vi "Start Needed uServices.vi"(8 "error in (no error)":errorcluster, 11 "Tamer in":refnum<class "Tamer.lvclass">) -> (0 "error out":errorcluster, 2 "All online?":bool, 3 "Tamer out":refnum<class "Tamer.lvclass">)   [LabVIEW 2020, in "TALOS.lvlib" / "Tamer.lvlib" / "Tamer.lvclass"]
uses:
  Tamer.lvclass
  Tamer.lvclass/Tamer.ctl
  Support VIs/Global Memory.vi
  Interfaces/FPGA Interface/FPGA Interface.lvclass
  TALOS.lvlib
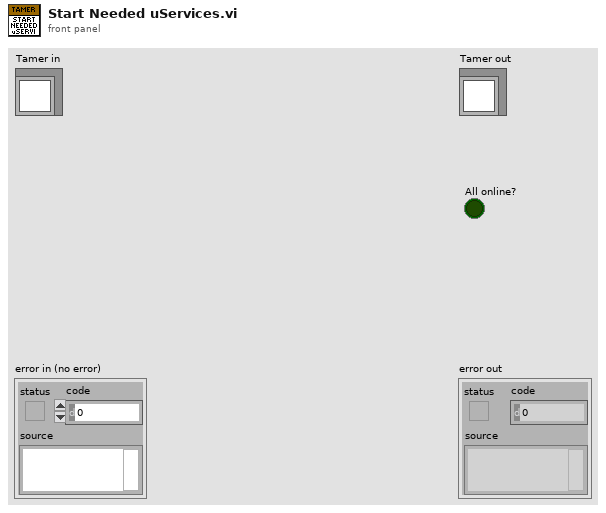
[diagram p1: front panel]
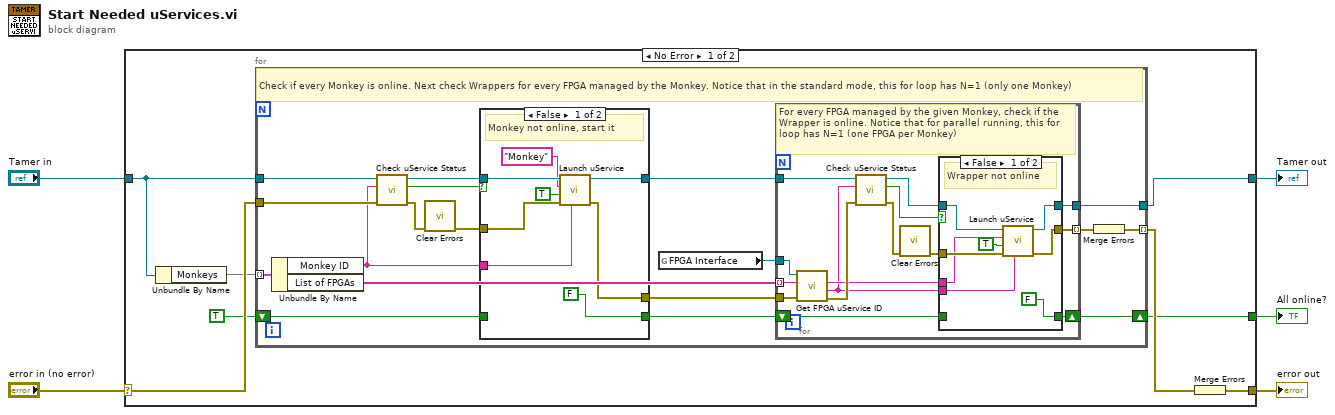
[diagram p0: block diagram]
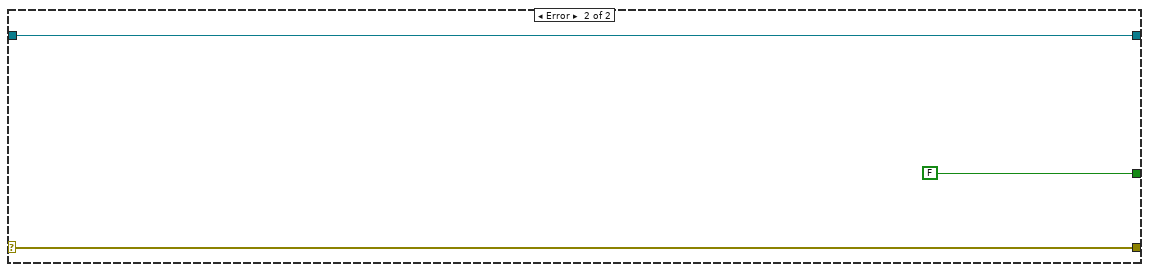
[diagram p4: hidden frame]
diagram:
  n1 = case shown="No Error" "error in (no error)" {
    selector: "error in (no error)" -> [w12 w71]
    tunnel: [w6 w71] -> w4
    tunnel: [w9 w70] -> w2
    tunnel: "Tamer in" -> [w10 w70]
    tunnel: [w7 FALSE] -> w1
    frame No Error {
      n2 = Unbundle By Name(w10) -> ("Monkeys"=w11:map{string, string[]})
      n3 = for {
        tunnel: w11 -> [w30] mode=indexing
        tunnel: w12 -> [w28]
        tunnel: w10 -> [w24]
        tunnel: [w21] -> w9
        tunnel: [w14] -> w13 mode=indexing
        shift-right: [w18] -> w7
        shift-left: TRUE -> [w20]
        # "Check if every Monkey is online. Next check Wrappers for every FPGA managed by the Monkey. Notice that in the standard mode, this for loop has N=1 (only one Monkey)"
        n4 = Unbundle By Name(w30) -> ("Monkey ID"=w25:string, "List of FPGAs"=w31:string[])
        n5 = call-dynamic "Check uService Status.vi"("error in (no error)"=w28, "uService ID"=w25, "Father of all uServices in"=w24) -> ("error out"=w29:errorcluster, "Online?"=w27:bool, "Father of all uServices out"=w26:refnum<class "Tamer.lvclass">)  [unwired: 5 in, 1 out]
        n6 = call <vilib>:"Clear Errors.vi"("error in (no error)"=w29) -> ("error out"=w23:errorcluster)  [unwired: 5 in, 1 out]
        n7 = case shown="False" w27 {
          tunnel: w26 -> [w38 w42]
          tunnel: w25 -> [w33 _]
          tunnel: [w37 w42] -> w22
          tunnel: w23 -> [w36 w41]
          tunnel: [w35 w41] -> w16
          tunnel: w20 -> [_ w40]
          tunnel: [FALSE w40] -> w19
          frame False {
            # "Monkey not online, start it"
            n8 = call-dynamic "Launch uService.vi"("uService ID (optional)"=w33, "error in (no error)"=w36, "GUI?"=TRUE, "Class Name"="Monkey", "Father of all uServices in"=w38) -> ("error out"=w35:errorcluster, "Father of all uServices out"=w37:refnum<class "Tamer.lvclass">)  [unwired: 5 in]
          }
          frame True {
            # "Monkey already online"
          }
        }
        n9 = global read "Global Memory.vi" "FPGA Interface"() -> (w17:refnum<class "FPGA Interface.lvclass">)
        n10 = for {
          tunnel: w31 -> [w47] mode=indexing
          tunnel: w22 -> [w57]
          tunnel: [w52] -> w21
          tunnel: [w51] -> w15 mode=indexing
          shift-right: [w49] -> w18
          shift-left: w19 -> [w50]
          tunnel: w17 -> [w48]
          tunnel: w16 -> [w46]
          # "For every FPGA managed by the given Monkey, check if the Wrapper is online. Notice that for parallel running, this for loop has N=1 (one FPGA per Monkey)"
          n11 = call-dynamic "Get FPGA uService ID.vi"("error in"=w46, "FPGA Name"=w47, "FPGA Interface"=w48) -> ("error out"=w45:errorcluster, "uService ID"=w43:string, "uService Class Name"=w44:string)  [unwired: 4 in]
          n12 = call-dynamic "Check uService Status.vi"("error in (no error)"=w45, "uService ID"=w43, "Father of all uServices in"=w57) -> ("error out"=w56:errorcluster, "Online?"=w53:bool, "Father of all uServices out"=w54:refnum<class "Tamer.lvclass">)  [unwired: 5 in, 1 out]
          n13 = call <vilib>:"Clear Errors.vi"("error in (no error)"=w56) -> ("error out"=w55:errorcluster)  [unwired: 5 in, 1 out]
          n14 = case shown="False" w53 {
            tunnel: w55 -> [w64 w67]
            tunnel: w54 -> [w63 w68]
            tunnel: [w62 w68] -> w52
            tunnel: [w61 w67] -> w51
            tunnel: w50 -> [_ w66]
            tunnel: [FALSE w66] -> w49
            tunnel: w44 -> [w59 _]
            tunnel: w43 -> [w58 _]
            frame False {
              # "Wrapper not online"
              n15 = call-dynamic "Launch uService.vi"("uService ID (optional)"=w58, "error in (no error)"=w64, "GUI?"=TRUE, "Class Name"=w59, "Father of all uServices in"=w63) -> ("error out"=w61:errorcluster, "Father of all uServices out"=w62:refnum<class "Tamer.lvclass">)  [unwired: 5 in]
            }
            frame True {
              # "Wrapper is online"
            }
          }
        }
        n16 = Merge Errors(w15) -> (w14:errorcluster)
      }
      n17 = Merge Errors(w13) -> (w6:errorcluster)
    }
    frame Error {
    }
  }
  "error out" <- w4
  "Tamer out" <- w2
  "All online?" <- w1
